vi "convert UTM to Pixels.vi"(8 "UTM position of Boat":T1 {"North" format="%#_10f"; "East" format="%#_8f"}, 9 "Bottum Right Pixel UTM":T1 {"North" format="%#_10f"; "East" format="%#_8f"}, 10 "Top Left Pixel UTM":T1 {"North" format="%#_10f"; "East" format="%#_8f"}, 11 "Map in":T2) -> (0 "Boat Outside Img":bool, 3 "Position":cluster{"X":i32, "Y":i32})   [LabVIEW 2013]
uses:
  <vilib>/vision/Image Controls.llb/IMAQ Image.ctl
  cRIO_Code/Data/TypeDefs/UTM Location.ctl
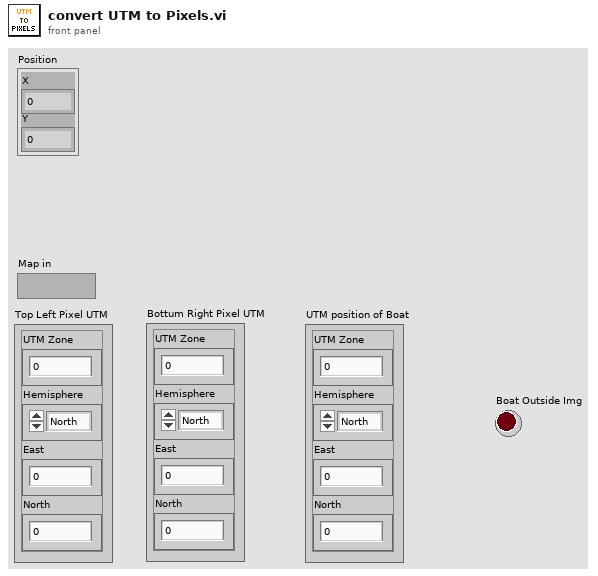
[diagram p1: front panel]
types:
  T1 = typedef "UTM Location.ctl" = cluster{"UTM Zone":dbl, "Hemisphere":enum16{"North", "South"}, "East":dbl, "North":dbl}
  T2 = typedef "IMAQ Image.ctl" = refnum<image>
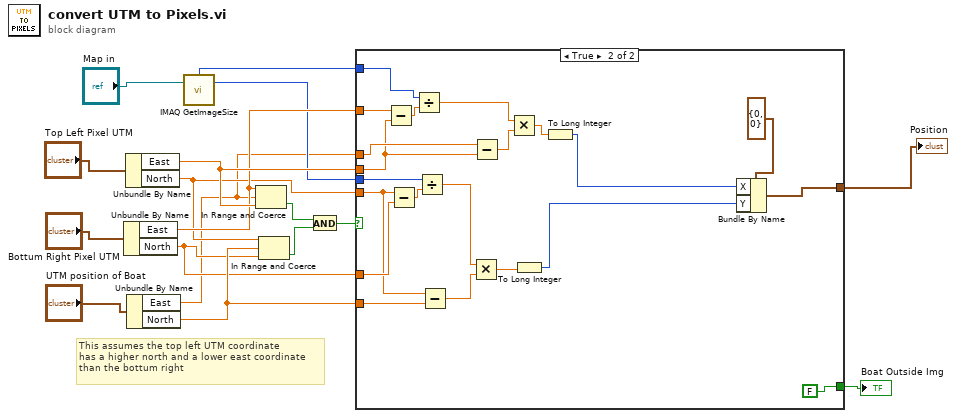
[diagram p0: block diagram]
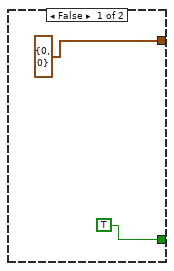
[diagram p2: hidden frame]
diagram:
  # "This assumes the top left UTM coordinate\nhas a higher north and a lower east coordinate\nthan the bottum right"
  n1 = Unbundle By Name("Bottum Right Pixel UTM") -> ("East"=w6:dbl, "North"=w3:dbl)
  n2 = Unbundle By Name("Top Left Pixel UTM") -> ("East"=w7:dbl, "North"=w4:dbl)
  n3 = Unbundle By Name("UTM position of Boat") -> ("East"=w2:dbl, "North"=w9:dbl)
  n4 = call "IMAQ GetImageSize"("Image"="Map in") -> ("Y Resolution"=w5:i32, "X Resolution"=w8:i32)  [unwired: 3 in, 1 out]
  n5 = In Range and Coerce(upper limit=w6, x=w2, lower limit=w7) -> (In Range?=w13:bool)  [unwired: 1 out]
  n6 = In Range and Coerce(upper limit=w4, x=w9, lower limit=w3) -> (In Range?=w12:bool)  [unwired: 1 out]
  n7 = And(x=w13, y=w12) -> (x .and. y?=w11:bool)
  n8 = case shown="True" w11 {
    tunnel: [TRUE FALSE] -> w10
    tunnel: w9 -> [_ w39]
    tunnel: w8 -> [_ w37]
    tunnel: w7 -> [_ w20]
    tunnel: w6 -> [_ w28]
    tunnel: w5 -> [_ w35]
    tunnel: w4 -> [_ w27]
    tunnel: w3 -> [_ w34]
    tunnel: w2 -> [_ w21]
    tunnel: [cluster{"X":i32, "Y":i32} {"X"=0, "Y"=0} ("Position 2") w24] -> w1
    frame False {
    }
    frame True {
      n9 = Subtract(x=w28, y=w20) -> (x-y=w38:dbl)
      n10 = Subtract(x=w27, y=w34) -> (x-y=w36:dbl)
      n11 = Divide(x=w37, y=w38) -> (x/y=w29:dbl)
      n12 = Divide(x=w35, y=w36) -> (x/y=w32:dbl)
      n13 = Subtract(x=w27, y=w39) -> (x-y=w33:dbl)
      n14 = Multiply(x=w32, y=w33) -> (x*y=w31:dbl)
      n15 = Subtract(x=w21, y=w20) -> (x-y=w30:dbl)
      n16 = Multiply(x=w29, y=w30) -> (x*y=w26:dbl)
      n17 = To Long Integer(number=w31) -> (32bit integer=w23:i32)
      n18 = To Long Integer(number=w26) -> (32bit integer=w22:i32)
      n19 = Bundle By Name(cluster=cluster{"X":i32, "Y":i32} {"X"=0, "Y"=0} ("Position 2"), "X"=w22, "Y"=w23) -> (w24:cluster{"X":i32, "Y":i32})
    }
  }
  "Boat Outside Img" <- w10
  "Position" <- w1
